vi "Acquire.vi"(8 "error in (no error)":errorcluster, 9 "Initialize":bool, 10 "Reply to":refnum<class "Result Reply Msg.lvclass">, 11 "Instrument Recorder in":refnum<class "Instrument Recorder.lvclass">) -> (0 "error out":errorcluster, 3 "Instrument Recorder out":refnum<class "Instrument Recorder.lvclass">)   [LabVIEW 2015, in "Instrument Recorder.lvclass"]
uses:
  Instrument Recorder.lvclass
  Measure Object Messages/Result Reply Msg/Result Reply Msg.lvclass
  Measure Object/Measure Object.lvclass
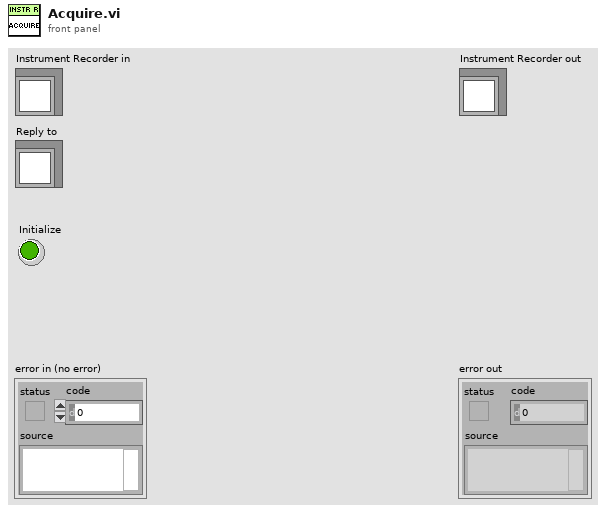
[diagram p1: front panel]
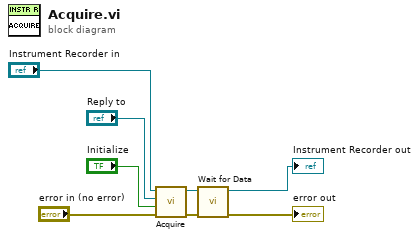
[diagram p0: block diagram]
diagram:
  n1 = call-parent "Acquire.vi"("error in (no error)"="error in (no error)", "Initialize"="Initialize", "Reply to"="Reply to", "Measure Object in"="Instrument Recorder in") -> ("error out"=w4:errorcluster, "Measure Object out"=w3:refnum<class "Instrument Recorder.lvclass">)  [unwired: 6 in]
  n2 = call-dynamic "Wait for Data.vi"("error in (no error)"=w4, "Instrument Recorder in"=w3) -> ("error out"=→"error out":errorcluster, "Instrument Recorder out"=→"Instrument Recorder out":refnum<class "Instrument Recorder.lvclass">)  [unwired: 8 in]
